vi "CRYDataView Docking Process.vi"(8 "DataView Index":i32, 9 "Start Pos":T1, 11 "Mouse Pos":T1) -> (3 "StartPositin Out":T1)   [LabVIEW 2013]
uses:
  CRYNew View Global.vi
  SubVI/CRYMain Sub Window Global.vi
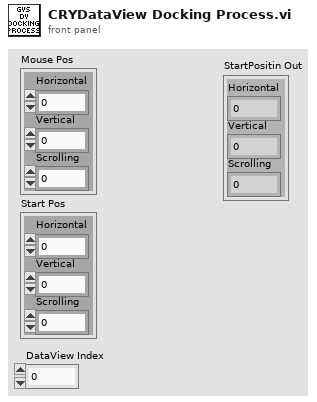
[diagram p1: front panel]
types:
  T1 = cluster{"Horizontal":i32, "Vertical":i32, "Scrolling":i32}
  T2 = typedef "Graph Main Info Cluster.ctl" = cluster{"Selected_BarIdx":i32, "Selected_PanelIdx":i32, "Graph Main VIRef":refnum<vi>, "ToolBarClick":bool, "Spliter Ref Array":refnum<vi>[], "Panel Ref Array":refnum<vi>[], "Spliter_matrix":i32[][], "Panel_matrix":i32[][], "child_spliterIdx_matrix":i32[][], "split_pos_matrix":i32[][], "Title State":bool, "sQueueName":string, "Frame nID":i32, "Graph VIRef Array":cluster{"Graph VIRef":refnum<vi>, "Panel Idx":i32, "Frame VIRef":refnum<vi>, "Icon Ring":i32, "Graph Type":string}[], "View Type":string}
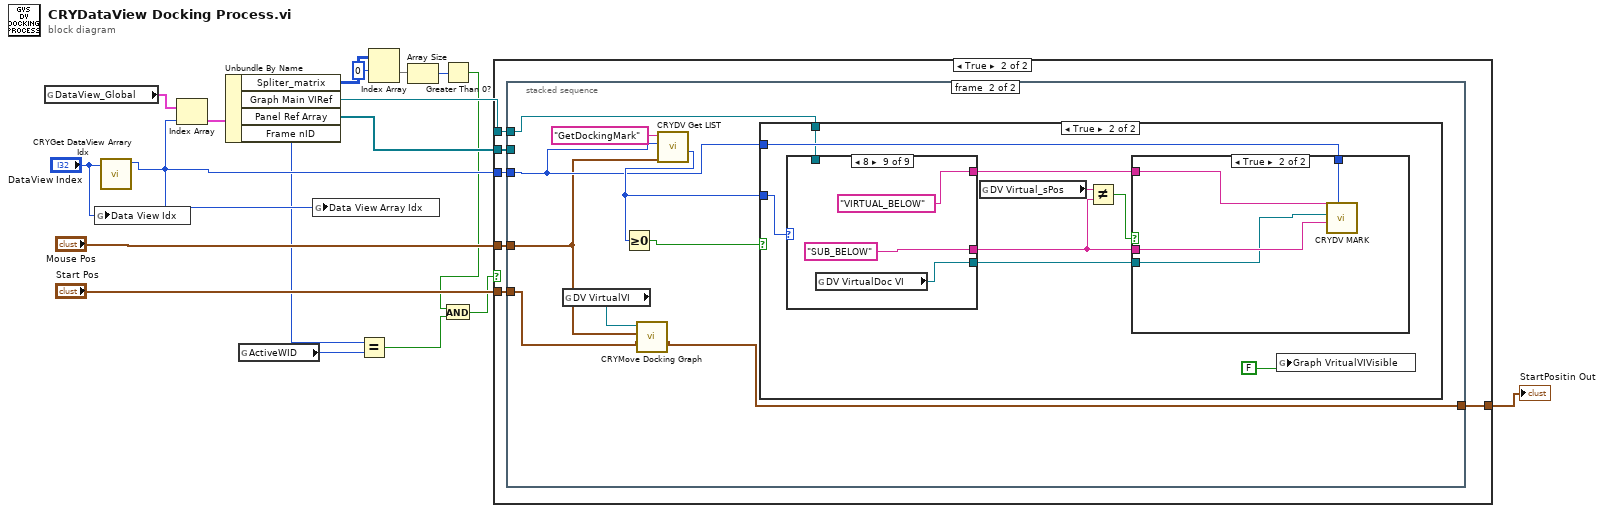
[diagram p0: block diagram]
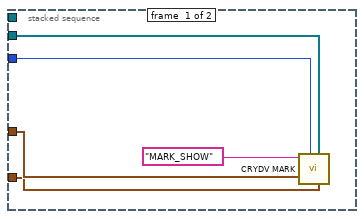
[diagram p3: hidden frame]
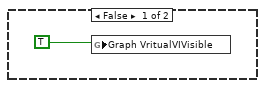
[diagram p4: hidden frame]
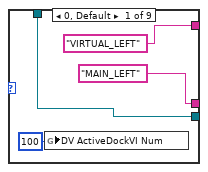
[diagram p6: hidden frame]
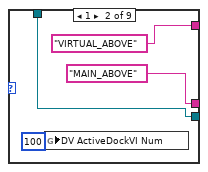
[diagram p7: hidden frame]
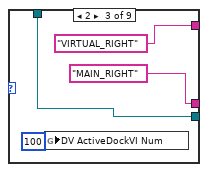
[diagram p8: hidden frame]
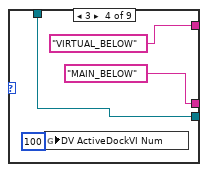
[diagram p9: hidden frame]
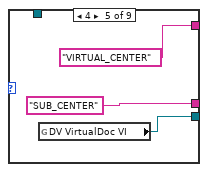
[diagram p10: hidden frame]
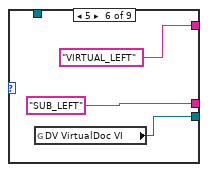
[diagram p11: hidden frame]
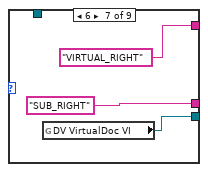
[diagram p12: hidden frame]
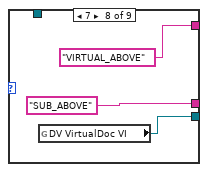
[diagram p13: hidden frame]
diagram:
  n1 = global read "CRYNew View Global.vi" "DataView_Global"() -> (w17:T2[])
  n2 = global write "CRYNew View Global.vi" "Data View Idx"("DataView Index") -> ()
  n3 = call "CRYGet DataView Arrary Idx.vi"("DataView Idx In"="DataView Index") -> ("DataView Arrary Idx out"=w7:i32)  [unwired: 10 in]
  n4 = Index Array(array=w17, index=w7) -> (element=w16:T2)
  n5 = Unbundle By Name(w16) -> ("Spliter_matrix"=w13:i32[][], "Graph Main VIRef"=w14:refnum<vi>, "Panel Ref Array"=w15:refnum<vi>[], "Frame nID"=w4:i32)
  n6 = global read "CRYMain Sub Window Global.vi" "ActiveWID"() -> (w5:i32)
  n7 = global write "CRYNew View Global.vi" "Data View Array Idx"(w7) -> ()
  n8 = Equal?(x=w4, y=w5) -> (x = y?=w2:bool)
  n9 = Index Array(array=w13, index (row)=0) -> (element=w11:i32[])  [unwired: 1 in]
  n10 = Array Size(array=w11) -> (size(s)=w10:i32)
  n11 = Greater Than 0?(x=w10) -> (x > 0?=w3:bool)
  n12 = And(x=w3, y=w2) -> (x .and. y?=w1:bool)
  n13 = case shown="True" w1 {
    tunnel: "Mouse Pos" -> [_ w25]
    tunnel: w7 -> [_ w24]
    tunnel: w15 -> [_ w23]
    tunnel: w14 -> [_ w22]
    tunnel: "Start Pos" -> [w19 w21]
    tunnel: [w19 w20] -> w9
    frame False {
    }
    frame True {
      n14 = stacked-sequence {
        tunnel: w25 -> [w27 w34]
        tunnel: w24 -> [w29 w35]
        tunnel: w23 -> [w28 _]
        tunnel: w22 -> [_ w36]
        tunnel: w21 -> [w26 w33]
        tunnel: [_ w31] -> w20
        frame #0 {
          n15 = call "CRYDV MARK.vi"("sAction"="MARK_SHOW", "MousePos"=w27, "DataView Array Index"=w29, "SubPanel array"=w28, "Start Pos In"=w26) -> ()  [unwired: 5 in, 1 out]
        }
        frame #1 {
          n16 = global read "CRYNew View Global.vi" "DV VirtualVI"() -> (w32:refnum<vi>)
          n17 = call "CRYMove Docking Graph.vi"("StartPositin In"=w33, "MousePositin In"=w34, "VI Ref In"=w32) -> ("StartPositin Out"=w31:T1)  [unwired: 6 in, 2 out]
          n18 = call "CRYDV Get LIST.vi"("sAction"="GetDockingMark", "DataView Array Index"=w35, "MousePos"=w34) -> ("nData_Out"=w37:i32)  [unwired: 4 in, 3 out]
          n19 = Greater Or Equal To 0?(x=w37) -> (x >= 0?=w38:bool)
          n20 = case shown="True" w38 {
            tunnel: w37 -> [_ w49]
            tunnel: w35 -> [_ w48]
            tunnel: w36 -> [_ w47]
            frame False {
              n21 = global write "CRYNew View Global.vi" "Graph VritualVIVisible"(TRUE ("VritualVIVisible")) -> ()
            }
            frame True {
              n22 = case shown="8" w49 {
                tunnel: ["MAIN_LEFT" ("sAction") "MAIN_ABOVE" ("sAction") "MAIN_RIGHT" ("sAction") "MAIN_BELOW" ("sAction") "SUB_CENTER" "SUB_LEFT" "SUB_RIGHT" "SUB_ABOVE" "SUB_BELOW"] -> w43
                tunnel: ["VIRTUAL_LEFT" ("sAction") "VIRTUAL_ABOVE" ("sAction") "VIRTUAL_RIGHT" ("sAction") "VIRTUAL_BELOW" ("sAction") "VIRTUAL_CENTER" "VIRTUAL_LEFT" "VIRTUAL_RIGHT" "VIRTUAL_ABOVE" "VIRTUAL_BELOW"] -> w44
                tunnel: w47 -> [w54 w58 w62 w66 _ _ _ _ _]
                tunnel: [w54 w58 w62 w66 w70 w73 w76 w79 w82] -> w41
                frame 0, Default {
                  n23 = global write "CRYNew View Global.vi" "DV ActiveDockVI Num"(100 ("ActiveDockVI Num")) -> ()
                }
                frame 1 {
                  n24 = global write "CRYNew View Global.vi" "DV ActiveDockVI Num"(100 ("ActiveDockVI Num")) -> ()
                }
                frame 2 {
                  n25 = global write "CRYNew View Global.vi" "DV ActiveDockVI Num"(100 ("ActiveDockVI Num")) -> ()
                }
                frame 3 {
                  n26 = global write "CRYNew View Global.vi" "DV ActiveDockVI Num"(100 ("ActiveDockVI Num")) -> ()
                }
                frame 4 {
                  n27 = global read "CRYNew View Global.vi" "DV VirtualDoc VI"() -> (w70:refnum<vi>)
                }
                frame 5 {
                  n28 = global read "CRYNew View Global.vi" "DV VirtualDoc VI"() -> (w73:refnum<vi>)
                }
                frame 6 {
                  n29 = global read "CRYNew View Global.vi" "DV VirtualDoc VI"() -> (w76:refnum<vi>)
                }
                frame 7 {
                  n30 = global read "CRYNew View Global.vi" "DV VirtualDoc VI"() -> (w79:refnum<vi>)
                }
                frame 8 {
                  n31 = global read "CRYNew View Global.vi" "DV VirtualDoc VI"() -> (w82:refnum<vi>)
                }
              }
              n32 = global read "CRYNew View Global.vi" "DV Virtual_sPos"() -> (w46:string)
              n33 = Not Equal?(x=w46, y=w43) -> (x != y?=w45:bool)
              n34 = case shown="True" w45 {
                tunnel: w44 -> [_ w53]
                tunnel: w43 -> [_ w52]
                tunnel: w48 -> [_ w51]
                tunnel: w41 -> [_ w50]
                frame False {
                }
                frame True {
                  n35 = call "CRYDV MARK.vi"("sAction"=w53, "mVritual_VIRef"=w50, "sData"=w52, "DataView Array Index"=w51) -> ()  [unwired: 6 in, 1 out]
                }
              }
              n36 = global write "CRYNew View Global.vi" "Graph VritualVIVisible"(FALSE ("VritualVIVisible")) -> ()
            }
          }
        }
      }
    }
  }
  "StartPositin Out" <- w9
